vi "Cleanup.vi"(8 "error in (no error)":errorcluster, 11 "Start High Pressure Wash in":refnum<class "Start High Pressure Wash.lvclass">) -> (0 "error out":errorcluster, 3 "Start High Pressure Wash out":refnum<class "Start High Pressure Wash.lvclass">)   [LabVIEW 2019, in "Start High Pressure Wash.lvclass"]
uses:
  <vilib>/gpm_packages/@cs/Car-wash/Source/Process Steps/Start High Pressure Wash/Start High Pressure Wash.lvclass
  <vilib>/gpm_packages/@cs/Car-wash/Source/iProcess Step Model/iProcess Step Model/iProcess Step Model.lvclass
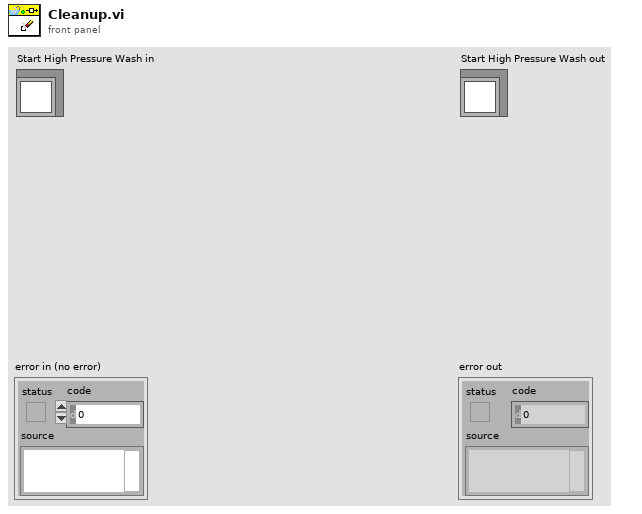
[diagram p1: front panel]
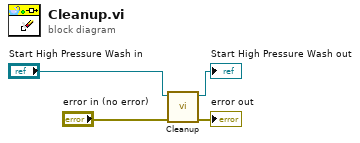
[diagram p0: block diagram]
diagram:
  n1 = call-parent "Cleanup.vi"("error in (no error)"="error in (no error)", "iProcess Step Model in"="Start High Pressure Wash in") -> ("error out"=→"error out":errorcluster, "iProcess Step Model out"=→"Start High Pressure Wash out":refnum<class "Start High Pressure Wash.lvclass">)  [unwired: 8 in]
